vi "SubVI_Mask_Grayscale&RGB #.vi"(5 "Image Register Name":string="untitled", 7 "Background Value":i32=255, 8 "Error in":errorcluster, 10 "ROI Descriptor":T2 {"Contours"."Type" items=["No Selection", "Point", "Line", "Rectangle", "Oval", "Polygon", "Freehand Region", "Annulus", "Unused2", "Unused3", "Broken Line", "Freehand Line", "Rotated Rectangle"]}, 11 "Image Src In":T1) -> (0 "Error out":errorcluster, 1 "Image Src Out":T1, 2 "ROI Descriptor out":T2 {"Contours"."Type" items=["No Selection", "Point", "Line", "Rectangle", "Oval", "Polygon", "Freehand Region", "Annulus", "Unused2", "Unused3", "Broken Line", "Freehand Line", "Rotated Rectangle"]}, 3 "Image Dst Out":T1)   [LabVIEW 2015]
uses:
  <vilib>/vision/Image Controls.llb/IMAQ Image.ctl
  <vilib>/vision/NI_Vision_Development_Module.lvlib
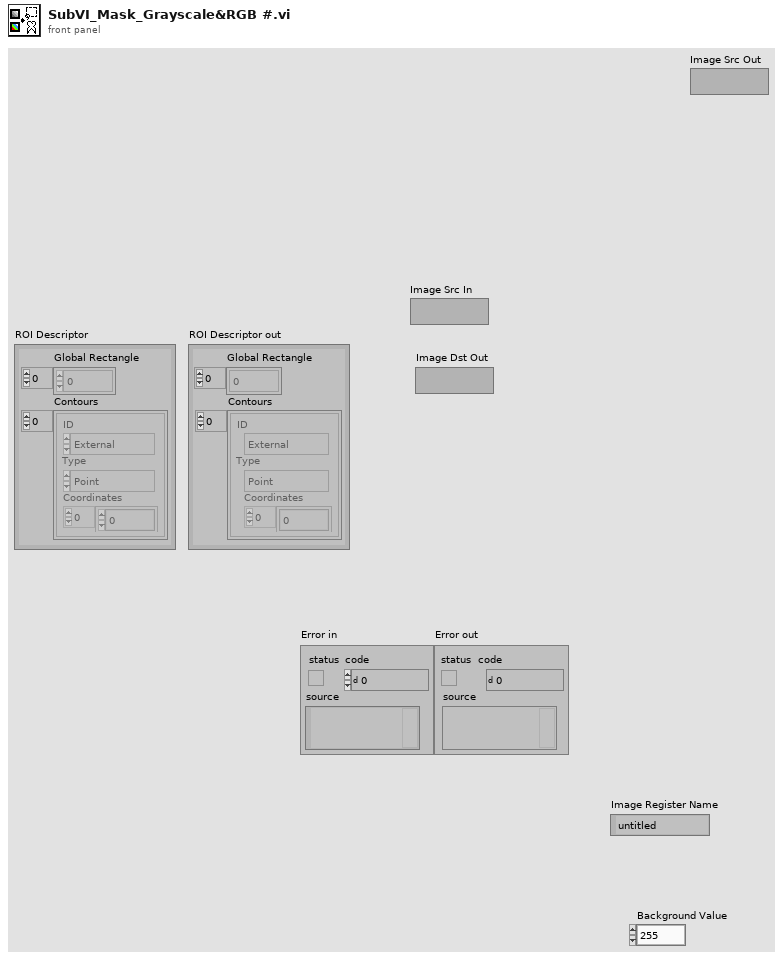
[diagram p1: front panel]
types:
  T1 = typedef "IMAQ Image.ctl" = refnum<image>
  T2 = typedef "ROI Descriptor" = cluster{"Global Rectangle":i32[], "Contours":cluster{"ID":enum32{"External", "Internal"}, "Type":u32, "Coordinates":i32[]}[]}
  T3 = cluster{"Origin":cluster{"X":sgl, "Y":sgl}, "Angle (deg)":sgl, "Axis Reference":u32}
  T4 = typedef "Image Type" = u32
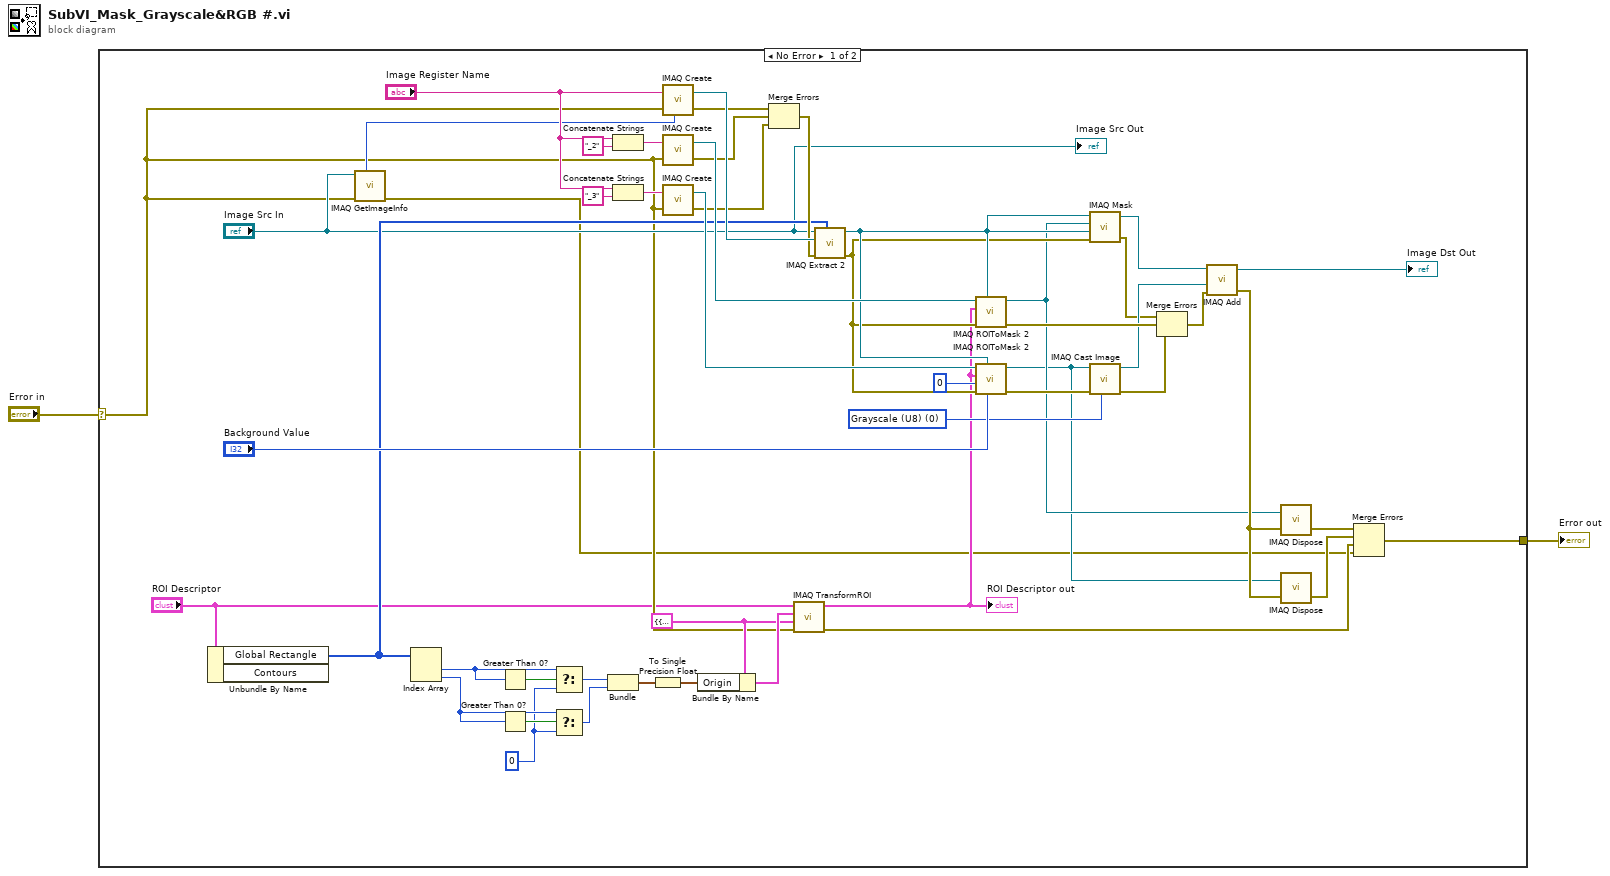
[diagram p0: block diagram]
diagram:
  n1 = case shown="No Error" "Error in" {
    selector: "Error in" -> [w5 w53]
    tunnel: [w22 w53] -> w2
    frame No Error {
      w14 = 0
      w17 = T3 {"Origin"={"X"=0.0, "Y"=0.0}, "Angle (deg)"=0.0, "Axis Reference"=0} ("Base Reference")
      w49 = T4 0 items=["Grayscale (U8)", "Grayscale (I16)", "Grayscale (SGL)", "Complex (CSG)", "RGB (U32)", "HSL (U32)", "RGB (U64)", "Grayscale (U16)"] ("Image Type")
      n2 = Unbundle By Name("ROI Descriptor") -> ("Global Rectangle"=w8:i32[])  [unwired: 1 out]
      n3 = call "IMAQ GetImageInfo"("error in (no error)"=w5, "Image"="Image Src In") -> ("error out"=w4:errorcluster, "Image Type"=w6:T4)  [unwired: 2 in, 6 out]
      n4 = Index Array(array=w8) -> (element #1=w21:i32, element #2=w20:i32)  [unwired: 2 in]
      n5 = Greater Than 0?(x=w21) -> (x > 0?=w16:bool)
      n6 = Greater Than 0?(x=w20) -> (x > 0?=w15:bool)
      n7 = Select(t=w21, s=w16, f=w14) -> (s? t:f=w13:i32)
      n8 = Select(t=w20, s=w15, f=w14) -> (s? t:f=w12:i32)
      n9 = Bundle(w13, w12) -> (w11:cluster{i32, i32})  [unwired: 1 in]
      n10 = Concatenate Strings("Image Register Name", "_2" ("string")) -> (w45:string)
      n11 = Concatenate Strings("Image Register Name", "_3" ("string")) -> (w43:string)
      n12 = To Single Precision Float(number=w11) -> (single precision float=w19:cluster{sgl, sgl})
      n13 = call "IMAQ Create"("Image Name"="Image Register Name", "Image Type"=w6, "error in (no error)"=w5) -> ("New Image"=w46:T1, "error out"=w39:errorcluster)  [unwired: 2 in]
      n14 = call "IMAQ Create"("Image Name"=w45, "error in (no error)"=w5) -> ("New Image"=w44:T1, "error out"=w38:errorcluster)  [unwired: 3 in]
      n15 = call "IMAQ Create"("Image Name"=w43, "error in (no error)"=w5) -> ("New Image"=w42:T1, "error out"=w37:errorcluster)  [unwired: 3 in]
      n16 = Bundle By Name(cluster=w17, "Origin"=w19) -> (w18:T3)
      n17 = Merge Errors(w39, w38, w37) -> (w36:errorcluster)
      n18 = call "IMAQ TransformROI"("error in (no error)"=w5, "New Reference"=w17, "Base Reference"=w18, "ROI Descriptor"="ROI Descriptor") -> ("error out"=w9:errorcluster, "ROI Descriptor out"=w10:T2)  [unwired: 6 in]
      "ROI Descriptor out" <- w10
      n19 = call "IMAQ Extract 2"("Optional Rectangle"=w8, "error in (no error)"=w36, "Image Dst"=w46, "Image Src"="Image Src In") -> ("error out"=w35:errorcluster, "Image Dst Out"=w41:T1)  [unwired: 6 in]
      n20 = call "IMAQ ROIToMask 2"("Image Model"=w41, "error in (no error)"=w35, "ROI Descriptor"=w10, "Image"=w44) -> ("error out"=w33:errorcluster, "Image Out"=w26:T1)  [unwired: 5 in, 1 out]
      n21 = call "IMAQ ROIToMask 2"("Background Value (0)"="Background Value", "Image Model"=w41, "error in (no error)"=w35, "Filling Value (255)"=0, "ROI Descriptor"=w10, "Image"=w42) -> ("error out"=w34:errorcluster, "Image Out"=w25:T1)  [unwired: 3 in, 1 out]
      n22 = call "IMAQ Mask"("error in (no error)"=w35, "Image Dst"=w41, "Image Mask"=w26, "Image Src"=w41) -> ("error out"=w28:errorcluster, "Image Dst Out"=w50:T1)  [unwired: 1 out]
      n23 = call "IMAQ Cast Image"("Image Type"=w49, "error in (no error)"=w34, "Image Src"=w25) -> ("error out"=w32:errorcluster, "Image Dst Out"=w30:T1)  [unwired: 7 in]
      n24 = Merge Errors(w28, w33, w32) -> (w31:errorcluster)
      n25 = call "IMAQ Add"("Image Src A"=w50, "Image Src B"=w30, "error in (no error)"=w31) -> ("Image Dst Out"=→"Image Dst Out":T1, "error out"=w27:errorcluster)  [unwired: 4 in]
      n26 = call "IMAQ Dispose"("Image"=w26, "error in (no error)"=w27) -> ("error out"=w24:errorcluster)  [unwired: 4 in]
      n27 = call "IMAQ Dispose"("Image"=w25, "error in (no error)"=w27) -> ("error out"=w23:errorcluster)  [unwired: 4 in]
      n28 = Merge Errors(w24, w23, w9, w4) -> (w22:errorcluster)
      "Image Src Out" <- "Image Src In"
    }
    frame Error {
    }
  }
  "Error out" <- w2
